vi "Set Pixel Size in Tag Value.vi"(4 "Litt/BigEnd":bool, 6 "DirEntries":T2[](array[typedef]), 7 "Pixels per unit":T1, 8 "Image Data in":u8[](array[numeric])) -> (3 "Image Data out":u8[](array[numeric]))   [LabVIEW 2015, in "Tiff reader.lvlib"]
doc: "Sets the Pixel Size Tag in the Tiff file."
uses:
  Tiff reader.lvlib
  IFD Entry.ctl
  FieldTypes.ctl
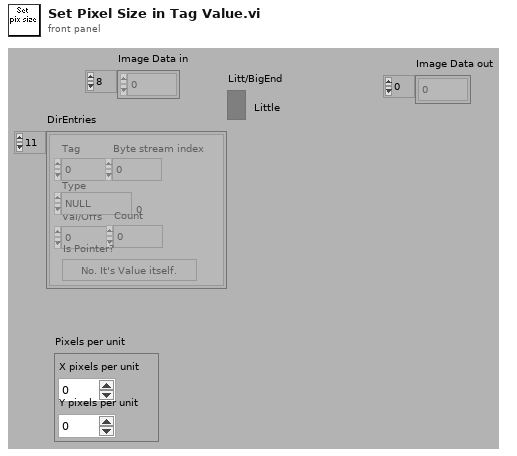
[diagram p1: front panel]
types:
  T1 = cluster{"X pixels per unit":dbl, "Y pixels per unit":dbl}
  T2 = typedef "Tiff reader.lvlib/IFD Entry.ctl" = cluster{"Tag":u16, "Type":T3, "Count":u32, "Val/Offs":u32, "Is Pointer?":bool, "Byte stream index":i32}
  T3 = typedef "Tiff reader.lvlib/FieldTypes.ctl" = enum16{"NULL", "U8", "ASCII7", "U16", "U32", "RATIONAL", "SByte(I8)", "Undef(8Bit)", "I16", "I32", "SRat(4B:4B)", "SGL(4Byte)", "DBL(8Byte)"}
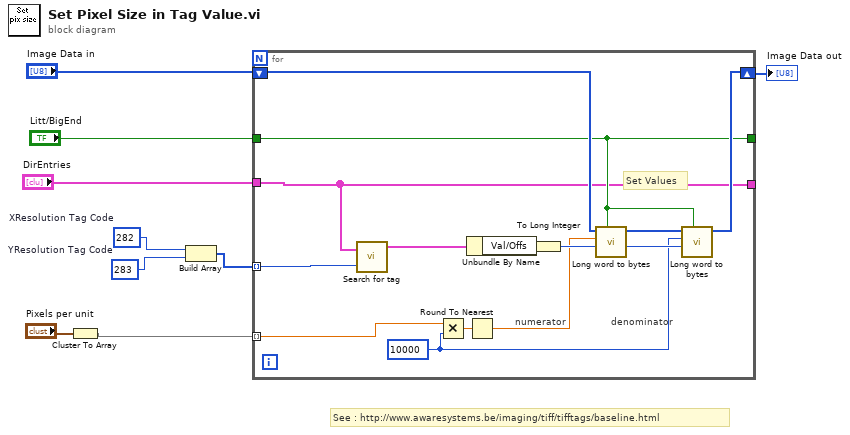
[diagram p0: block diagram]
diagram:
  w6 = u16 283  # YResolution Tag Code
  w3 = u16 282  # XResolution Tag Code
  # "See : http://www.awaresystems.be/imaging/tiff/tifftags/baseline.html"
  n1 = Cluster To Array(cluster="Pixels per unit") -> (array=w7:dbl[])
  n2 = Build Array(w3, w6) -> (w9:u16[])
  n3 = for {
    tunnel: "DirEntries" -> [w11]
    tunnel: w9 -> [w10] mode=indexing
    tunnel: "Litt/BigEnd" -> [w13]
    tunnel: w7 -> [w14] mode=indexing
    shift-right: [w15] -> w1
    shift-left: "Image Data in" -> [w16]
    tunnel: [w13] -> _
    tunnel: [w11] -> _
    w18 = u32 10000
    # "denominator"
    # "numerator"
    # "Set Values"
    n4 = call "Search for tag.vi"("Directory"=w11, "Tag"=w10) -> ("Tag found"=w12:T2)  [unwired: 2 out]
    n5 = Multiply(x=w14, y=w18) -> (x*y=w22:dbl)
    n6 = Unbundle By Name(w12) -> ("Val/Offs"=w23:u32)
    n7 = Round To Nearest(number=w22) -> (nearest integer value=w17:dbl)
    n8 = To Long Integer(number=w23) -> (32bit integer=w21:i32)
    n9 = call "Long word to bytes.vi"("Litt/BigEnd"=w13, "Index"=w21, "U32"=w17, "Image Data in"=w16) -> ("Index+4"=w19:i32, "Image Data out"=w20:u8[])  [unwired: 4 out]
    n10 = call "Long word to bytes.vi"("Litt/BigEnd"=w13, "Index"=w19, "U32"=w18, "Image Data in"=w20) -> ("Image Data out"=w15:u8[])  [unwired: 5 out]
  }
  "Image Data out" <- w1
